vi "Calculate no of Hist bins.vi"(0 "Mean":dbl, 1 "Standard Deviation":dbl, 2 "Time Trace":dbl[](array[numeric]), 3 "Shift Input":T1, 4 "Number of Bins per Sigma":dbl=50.0 format="%#_13g") -> (6 "Shift Output":T1)   [LabVIEW 2016]
uses:
  Controls/Shift_Cluster.ctl
  Globals/Meas_global.vi
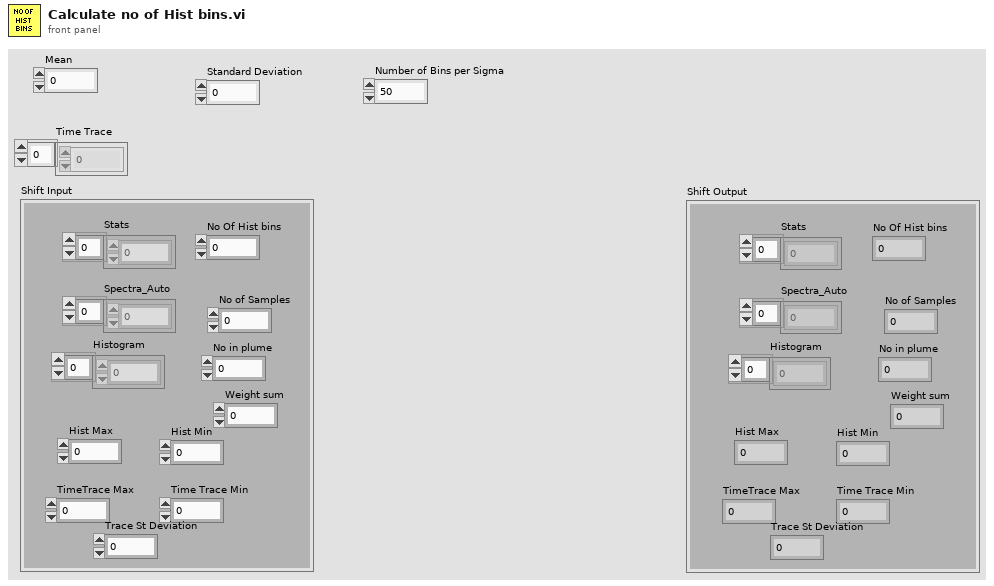
[diagram p1: front panel]
types:
  T1 = typedef "Shift_Cluster.ctl" = cluster{"Stats":dbl[], "Spectra_Auto":dbl[], "Histogram":dbl[], "Hist Max":dbl, "Hist Min":dbl, "No of Samples":i32, "No in plume":i32, "Weight sum":dbl, "No Of Hist bins":i32, "TimeTrace Max":dbl, "Time Trace Min":dbl, "Trace St Deviation":dbl}
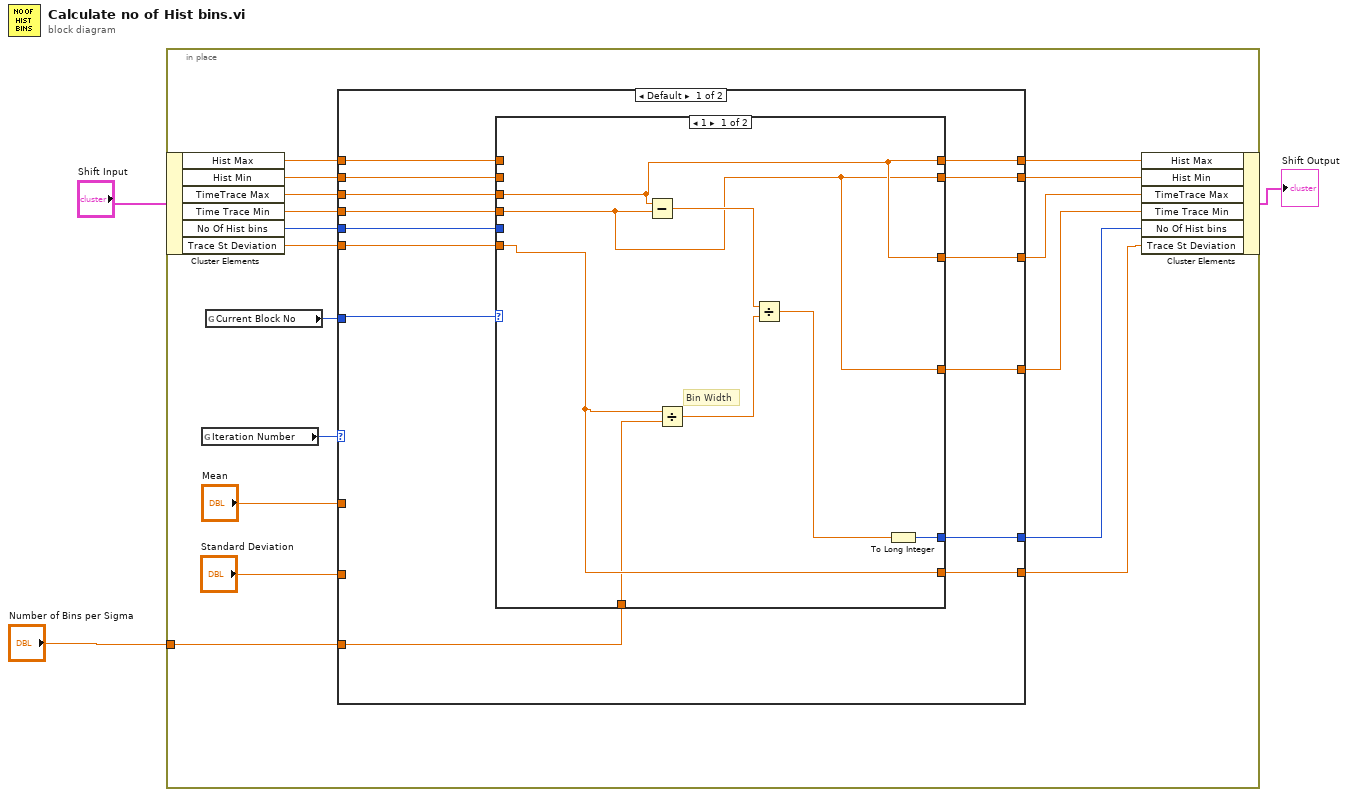
[diagram p0: block diagram]
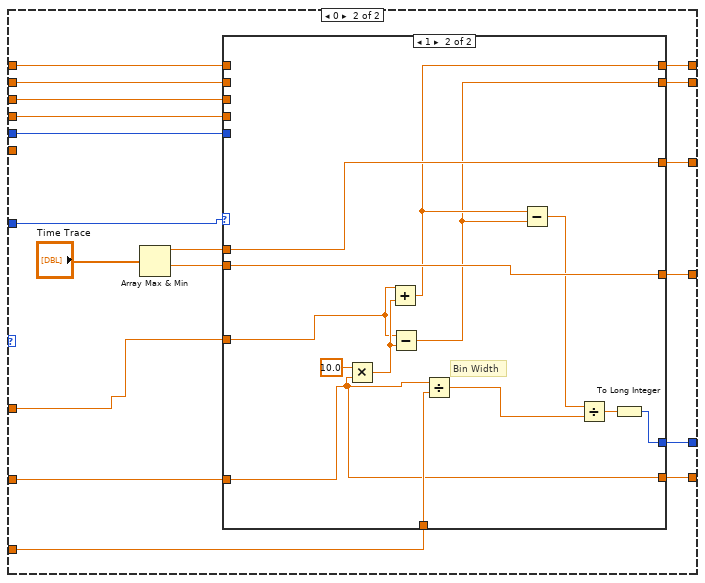
[diagram p3: hidden frame]
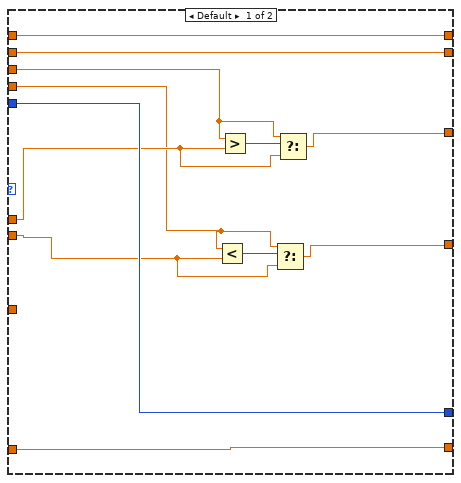
[diagram p4: hidden frame]
diagram:
  n1 = in-place {
    in-place-border: "Number of Bins per Sigma" -> [w6]
    n2 = in-place-cluster #1("Shift Input") -> ("Hist Max"=w13:dbl, "Hist Min"=w12:dbl, "TimeTrace Max"=w10:dbl, "Time Trace Min"=w9:dbl, "No Of Hist bins"=w11:i32, "Trace St Deviation"=w7:dbl)
    n3 = global read "Meas_global.vi" "Iteration Number"() -> (w20:i32)
    n4 = global read "Meas_global.vi" "Current Block No"() -> (w19:i32)
    n5 = case shown="Default" w20 {
      tunnel: w19 -> [w34 w65]
      tunnel: [w26 w64] -> w16
      tunnel: [w29 w63] -> w15
      tunnel: [w30 w60] -> w14
      tunnel: [w25 w59] -> w18
      tunnel: [w22 w58] -> w17
      tunnel: w13 -> [w24 w57]
      tunnel: w12 -> [w23 w56]
      tunnel: w11 -> [w31 w55]
      tunnel: w10 -> [w27 w54]
      tunnel: w9 -> [w28 w53]
      tunnel: [w33 w52] -> w8
      tunnel: w7 -> [w32 _]
      tunnel: w6 -> [w21 w51]
      tunnel: "Mean" -> [_ w50]
      tunnel: "Standard Deviation" -> [_ w49]
      frame Default {
        n6 = case shown="1" w34 {
          tunnel: [w38 w48] -> w33
          tunnel: w32 -> [w38 w48]
          tunnel: w31 -> [_ w47]
          tunnel: [w39 w47] -> w30
          tunnel: [w36 w46] -> w29
          tunnel: w28 -> [w36 w46]
          tunnel: w27 -> [w37 w45]
          tunnel: [w37 w45] -> w26
          tunnel: [w37 w44] -> w25
          tunnel: w24 -> [_ w44]
          tunnel: w23 -> [_ w43]
          tunnel: [w36 w43] -> w22
          tunnel: w21 -> [w35 _]
          frame 1 {
            # "Bin Width"
            n7 = Subtract(x=w37, y=w36) -> (x-y=w42:dbl)
            n8 = Divide(x=w38, y=w35) -> (x/y=w41:dbl)
            n9 = Divide(x=w42, y=w41) -> (x/y=w40:dbl)
            n10 = To Long Integer(number=w40) -> (32bit integer=w39:i32)
          }
          frame Default {
          }
        }
      }
      frame 0 {
        n11 = Array Max & Min(array="Time Trace") -> (max value=w62:dbl, min value=w61:dbl)  [unwired: 2 out]
        n12 = case shown="1" w65 {
          tunnel: [w74 w91] -> w64
          tunnel: [w70 w90] -> w63
          tunnel: w62 -> [w72 w91]
          tunnel: w61 -> [w68 w90]
          tunnel: [w76 w86] -> w60
          tunnel: [w78 w83] -> w59
          tunnel: [w77 w82] -> w58
          tunnel: w57 -> [w78 _]
          tunnel: w56 -> [w77 _]
          tunnel: w55 -> [w76 _]
          tunnel: w54 -> [w73 _]
          tunnel: w53 -> [w69 _]
          tunnel: [w67 w79] -> w52
          tunnel: w51 -> [_ w81]
          tunnel: w50 -> [_ w80]
          tunnel: w49 -> [w67 w79]
          frame Default {
            n13 = Less?(x=w69, y=w68) -> (x < y?=w71:bool)
            n14 = Greater?(x=w73, y=w72) -> (0:w75:bool)
            n15 = Select(t=w69, s=w71, f=w68) -> (s? t:f=w70:dbl)
            n16 = Select(t=w73, s=w75, f=w72) -> (s? t:f=w74:dbl)
          }
          frame 1 {
            # "Bin Width"
            n17 = Multiply(x=10.0, y=w79) -> (x*y=w84:dbl)
            n18 = Add(x=w80, y=w84) -> (x+y=w83:dbl)
            n19 = Subtract(x=w80, y=w84) -> (x-y=w82:dbl)
            n20 = Divide(x=w79, y=w81) -> (x/y=w88:dbl)
            n21 = Subtract(x=w83, y=w82) -> (x-y=w89:dbl)
            n22 = Divide(x=w89, y=w88) -> (x/y=w87:dbl)
            n23 = To Long Integer(number=w87) -> (32bit integer=w86:i32)
          }
        }
      }
    }
    n24 = in-place-cluster #1("Hist Max"=w18, "Hist Min"=w17, "TimeTrace Max"=w16, "Time Trace Min"=w15, "No Of Hist bins"=w14, "Trace St Deviation"=w8) -> (→"Shift Output":T1)
  }
